vi "Compute Registry Key.vi"(10 "SMO GUID":string, 11 "Registry's SecretKey":string) -> (3 "Registry Key":string)   [LabVIEW 2019, in "Registry-SMO.lvclass"]
doc: "JKI State Machine Objects (SMO) 1.3.0.56\nJKI - JKI\nCopyright (c) 2017, JKI"
uses:
  Registry-SMO.lvclass
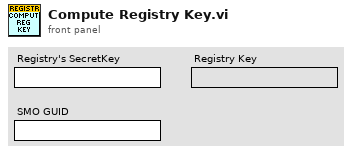
[diagram p1: front panel]
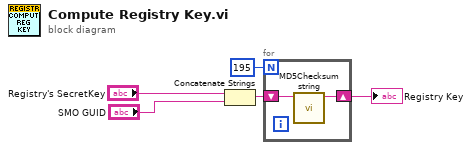
[diagram p0: block diagram]
diagram:
  n1 = Concatenate Strings("Registry's SecretKey", "SMO GUID") -> (w2:string)
  n2 = for {
    N: 195 -> [_]
    shift-right: [w6] -> w5
    shift-left: w2 -> [w7]
    n3 = call <vilib>:"MD5Checksum string.vi"("Message String"=w7) -> ("MD5 message-digest"=w6:string)  [unwired: 10 in]
  }
  "Registry Key" <- w5
